vi "template_labview.vi"() -> ()   [LabVIEW 2022 SP3]
uses:
  <vilib>/Utility/file.llb/Write Delimited Spreadsheet (string).vi
  <vilib>/Utility/file.llb/Read Delimited Spreadsheet (string).vi
panel:
  in  "read":bool
  out "all rows":string[][](array[string]) caption="所有行"
  in  "save":bool
  out "数组":string[][](array[string])
  in  "布尔":bool
  in  "数值":i32
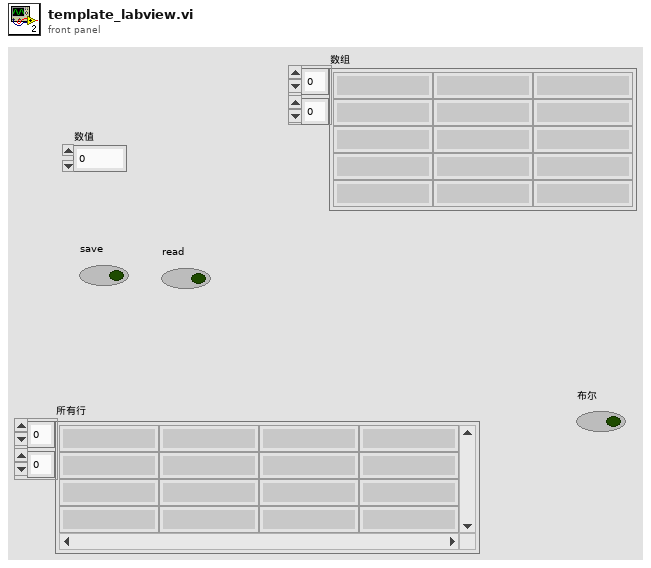
[diagram p1: front panel]
types:
  T1 = cluster{"Number":i32, "Path":path, "Array":string[][]}
  T2 = enum16{"open", "replace", "create", "open or create", "replace or create", "replace or create with confirmation"}
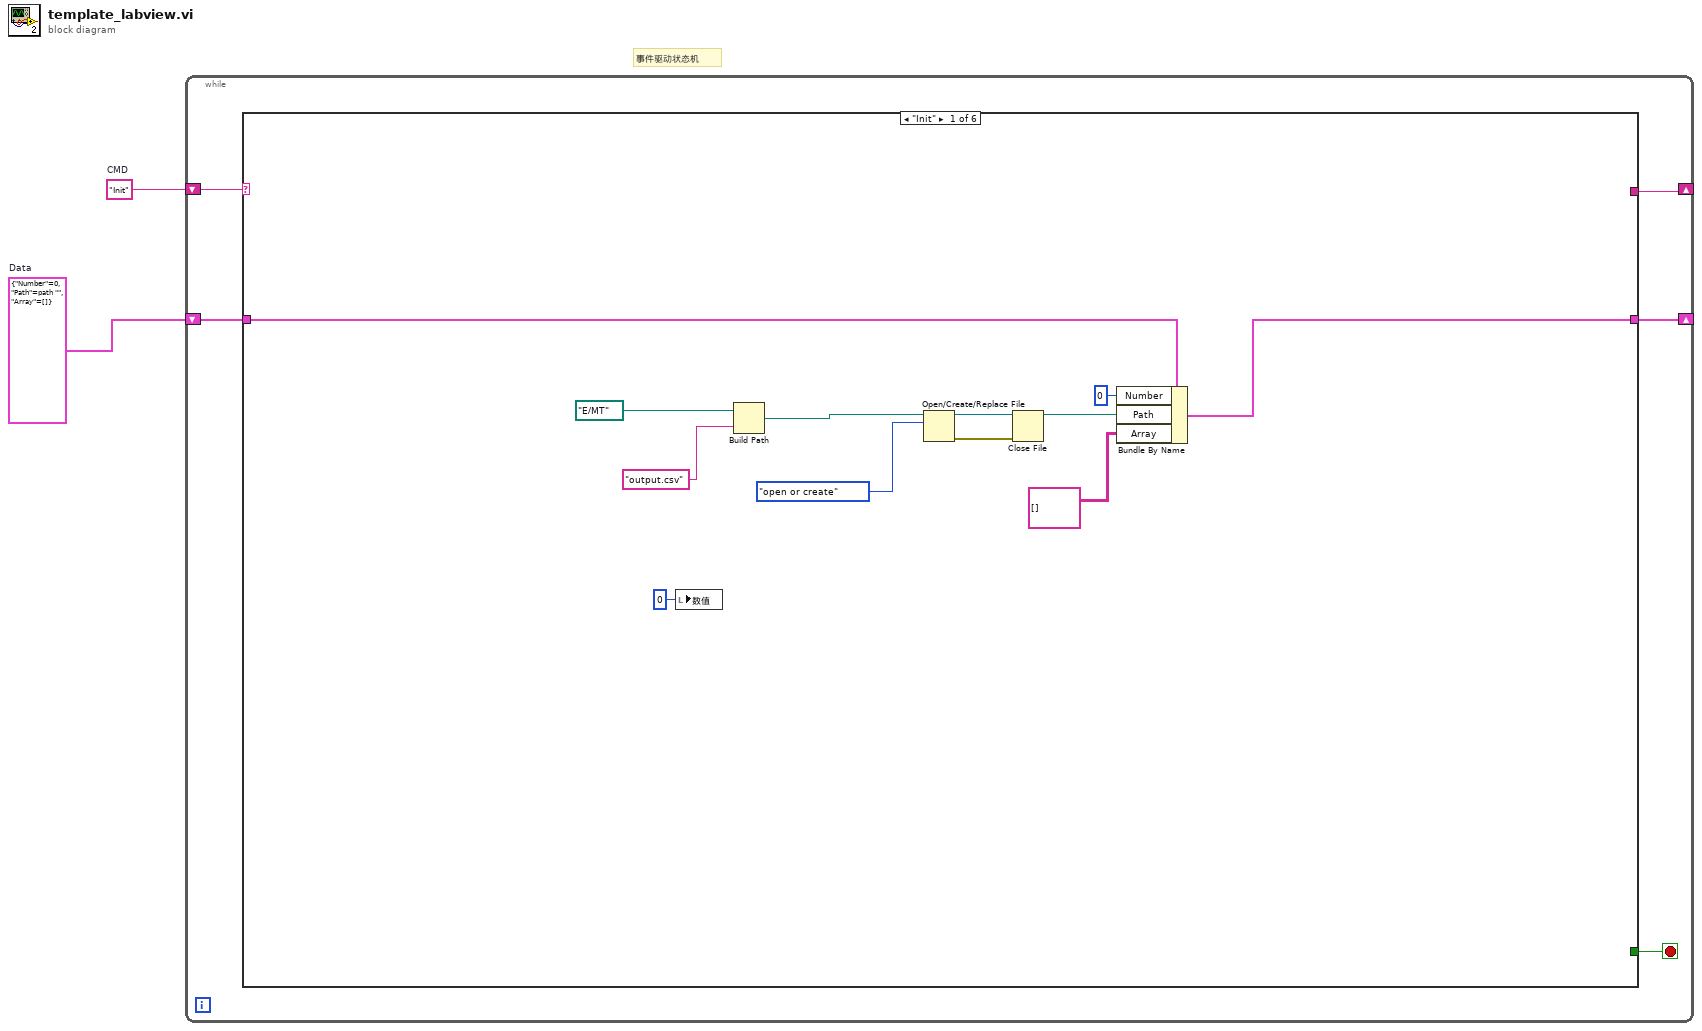
[diagram p0: block diagram]
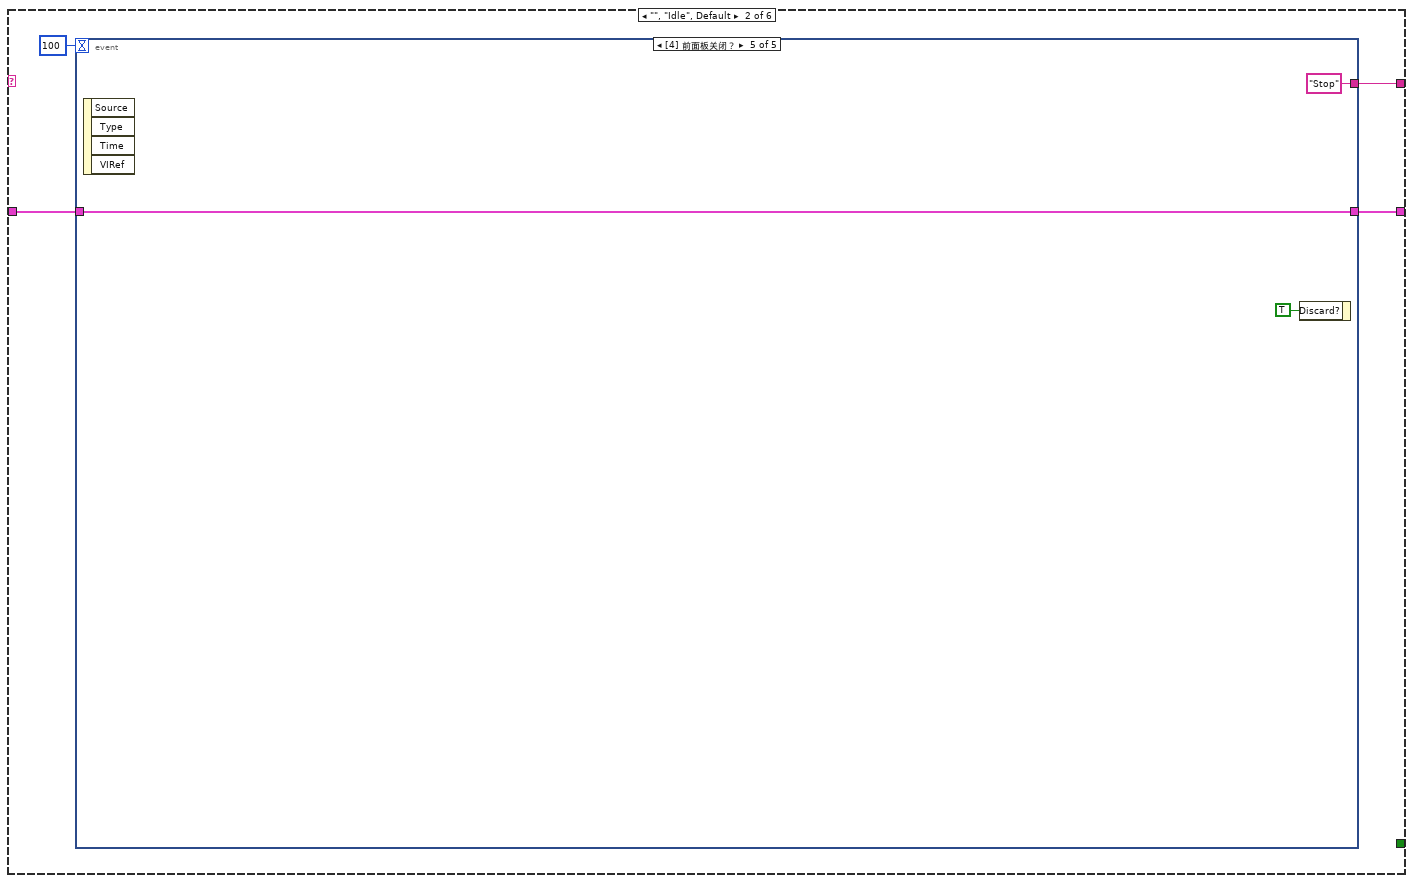
[diagram p2: hidden frame]
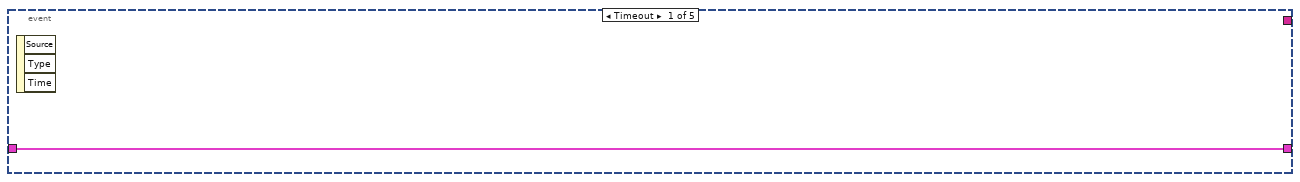
[diagram p3: hidden frame]
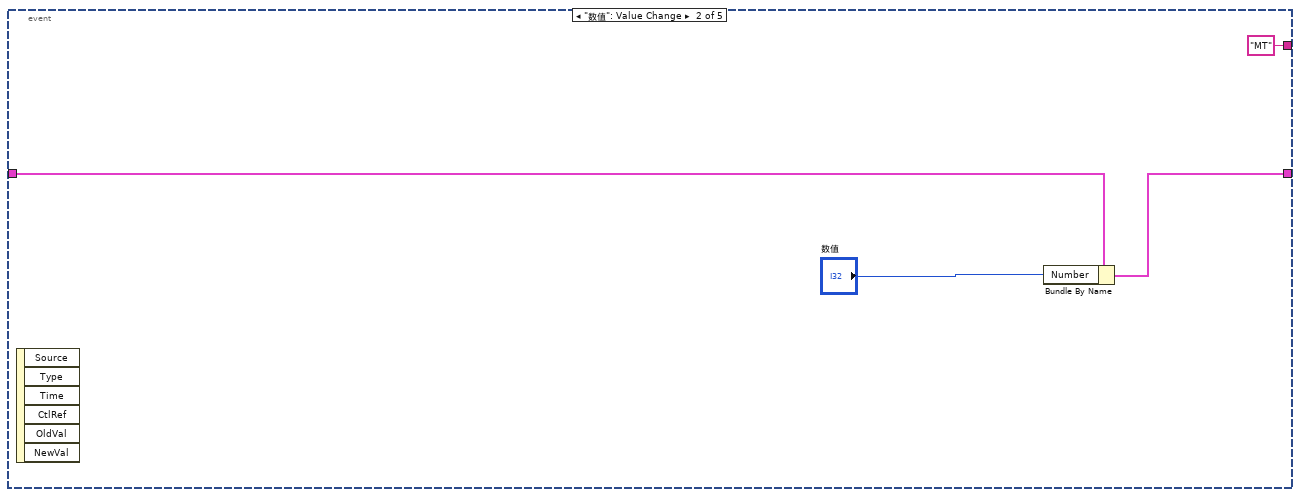
[diagram p4: hidden frame]
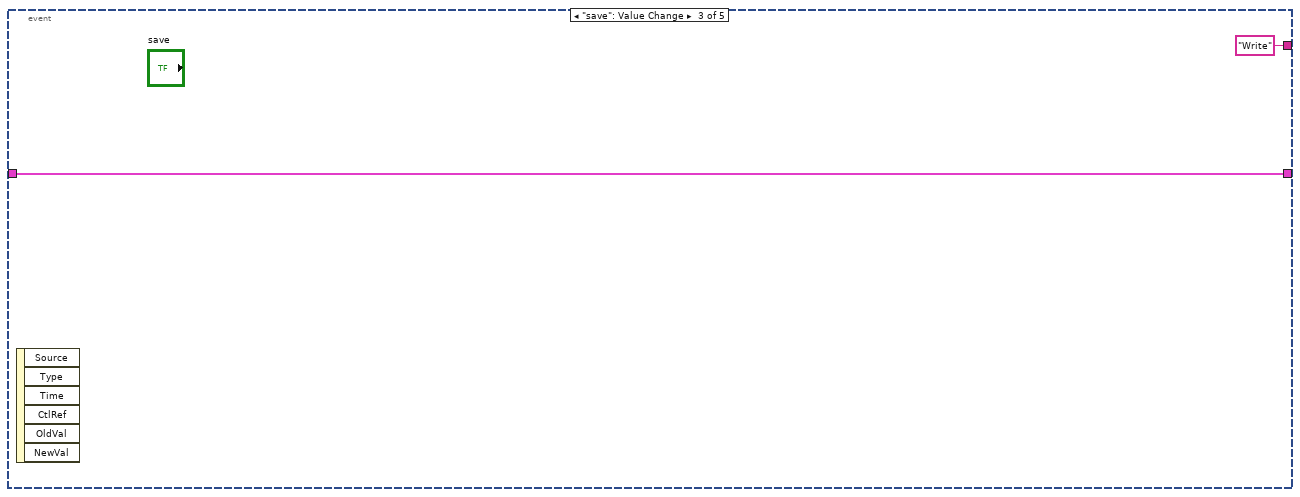
[diagram p5: hidden frame]
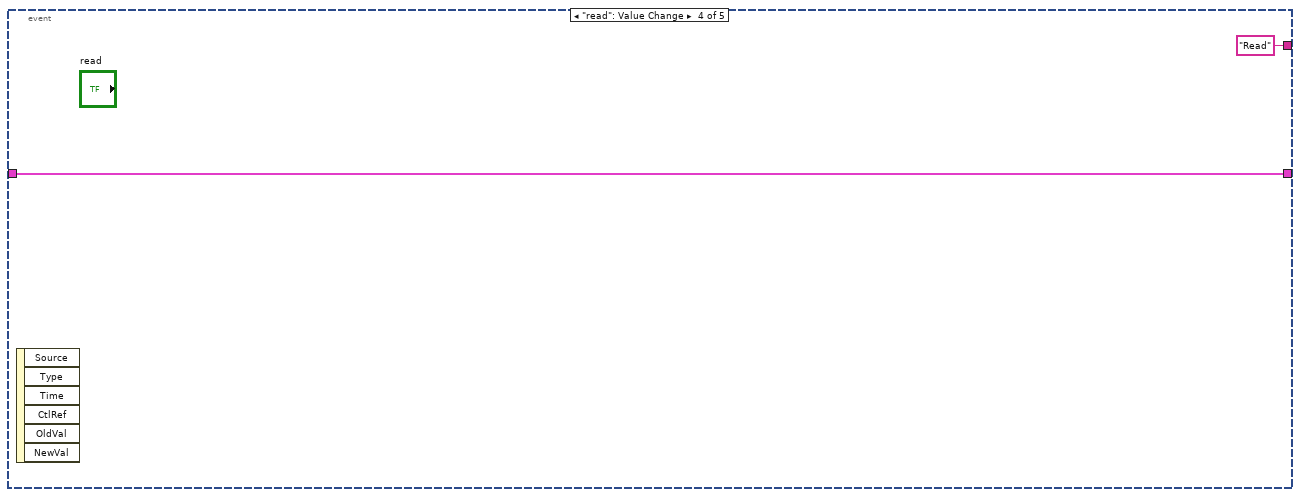
[diagram p6: hidden frame]
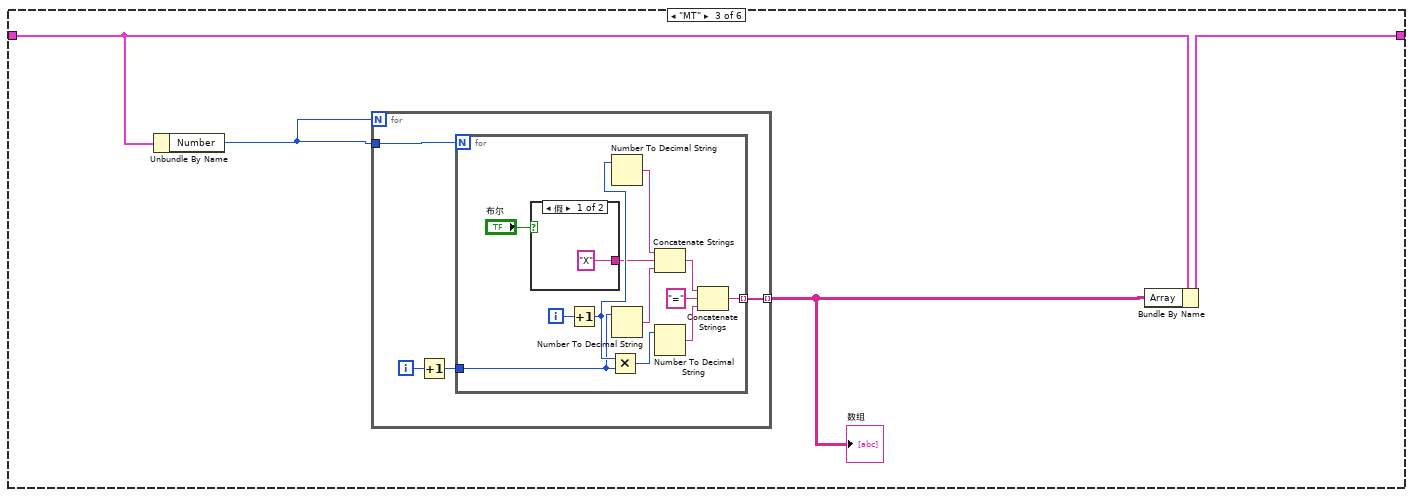
[diagram p7: hidden frame]
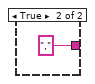
[diagram p8: hidden frame]
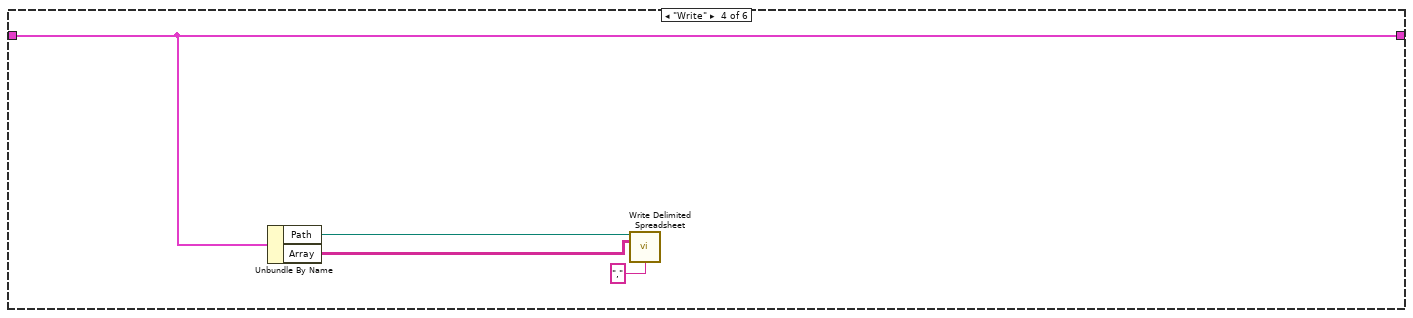
[diagram p9: hidden frame]
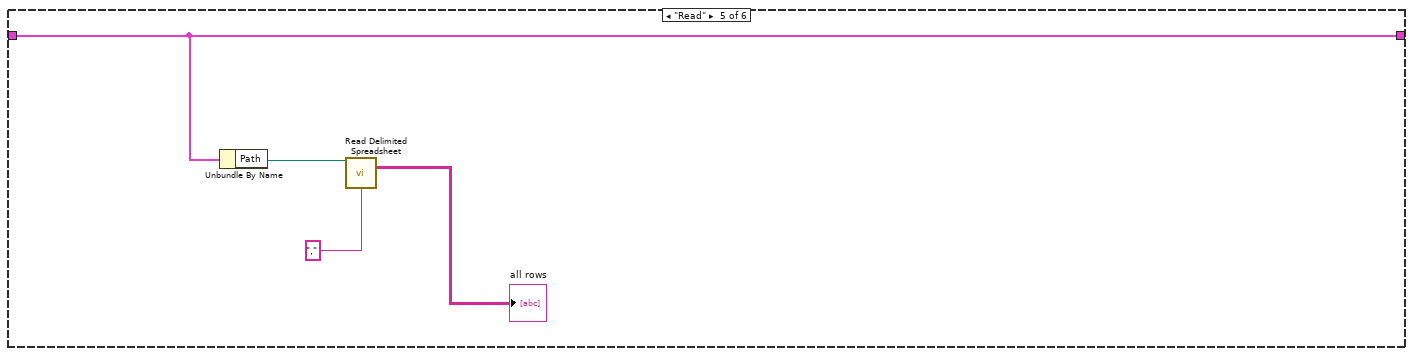
[diagram p10: hidden frame]
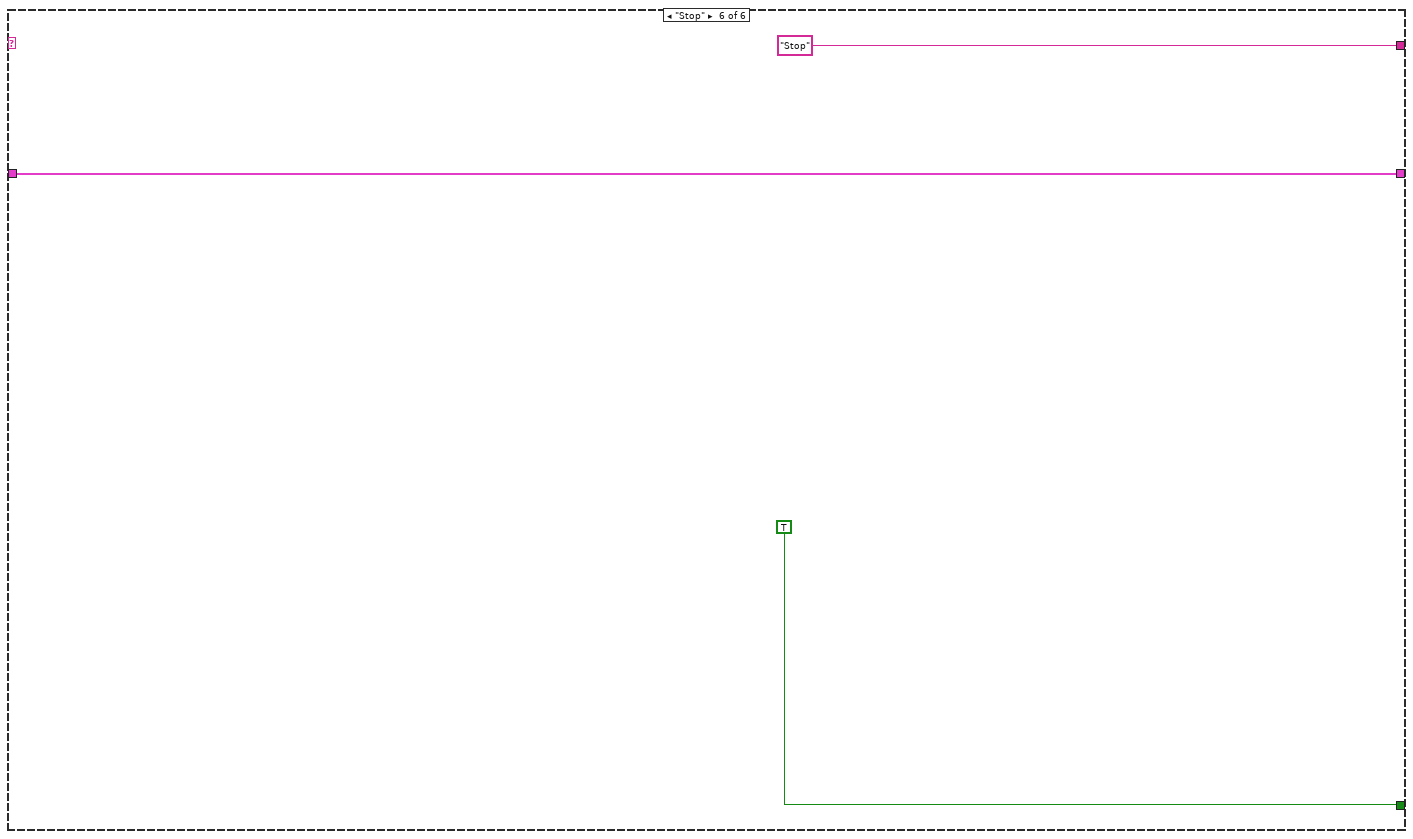
[diagram p11: hidden frame]
diagram:
  w1 = T1 {"Number"=0, "Path"=path "", "Array"=[]}  # Data
  w2 = "Init"  # CMD
  # "事件驱动状态机"
  n1 = while {
    shift-right: [w5] -> _
    shift-left: w2 -> [w7]
    shift-right: [w3] -> _
    shift-left: w1 -> [w4]
    stop <- w6 stop-if-true
    n2 = case shown="\"Init\"" w7 {
      tunnel: [_ _ _ _ _ TRUE] -> w6
      tunnel: [_ w22 _ _ _ "Stop"] -> w5
      tunnel: w4 -> [w19 w21 w39 w60 w65 w66]
      tunnel: [w18 w20 w37 w60 w65 w66] -> w3
      frame "Init" {
        n3 = local write "数值"(0 ("数值")) -> ()
        n4 = Build Path(base path=path "E:/MT" ("Path"), name or relative path="output.csv") -> (appended path=w13:path)
        n5 = Open/Create/Replace File(file path (use dialog)=w13, operation (0:open)=T2."open or create" ("操作(0:open)")) -> (refnum out=w12:refnum<file>, error out=w10:errorcluster)  [unwired: 4 in, 1 out]
        n6 = Close File(refnum=w12, error in=w10) -> (path=w11:path)  [unwired: 1 out]
        n7 = Bundle By Name(cluster=w19, "Number"=0, "Path"=w11, "Array"=string[][] []) -> (w18:T1)
      }
      frame "", "Idle", Default {
        n8 = event shown="[4] 前面板关闭？" {
          selector: _ -> [_ _ _ _ _]
          dyn-events: _ -> [_ _ _ _ _]
          timeout: 100 -> [_ _ _ _ _]
          tunnel: [_ "MT" "Write" "Read" "Stop"] -> w22
          tunnel: w21 -> [w24 w28 w30 w32 w33]
          tunnel: [w24 w27 w30 w32 w33] -> w20
          event Timeout {
            n9 = event-data() -> ()  [unwired: 1 in, 3 out]
          }
          event "数值": Value Change {
            n10 = event-data() -> ()  [unwired: 1 in, 6 out]
            n11 = Bundle By Name(cluster=w28, "Number"="数值") -> (w27:T1)
          }
          event "save": Value Change {
            n12 = event-data() -> ()  [unwired: 1 in, 6 out]
          }
          event "read": Value Change {
            n13 = event-data() -> ()  [unwired: 1 in, 6 out]
          }
          event Panel Close? {
            n14 = event-data() -> ()  [unwired: 1 in, 4 out]
            n15 = event-data("Discard?"=TRUE ("放弃？")) -> ()  [unwired: 1 in, 1 out]
          }
        }
      }
      frame "MT" {
        n16 = Unbundle By Name(w39) -> ("Number"=w38:i32)
        n17 = for {
          N: w38 -> [_]
          tunnel: w38 -> [w43]
          tunnel: [w40] -> w36 mode=indexing
          i -> [w42]
          n18 = Increment(x=w42) -> (x+1=w41:i32)
          n19 = for {
            N: w43 -> [_]
            tunnel: w41 -> [w52]
            tunnel: [w44] -> w40 mode=indexing
            i -> [w54]
            n20 = case shown="假" "布尔" {
              tunnel: ["X" ","] -> w51
              frame False {
              }
              frame True {
              }
            }
            n21 = Increment(x=w54) -> (x+1=w53:i32)
            n22 = Multiply(x=w53, y=w52) -> (x*y=w46:i32)
            n23 = Number To Decimal String(number=w53) -> (decimal integer string=w50:string)  [unwired: 1 in]
            n24 = Number To Decimal String(number=w52) -> (decimal integer string=w49:string)  [unwired: 1 in]
            n25 = Concatenate Strings(w50, w51, w49) -> (w47:string)
            n26 = Number To Decimal String(number=w46) -> (decimal integer string=w45:string)  [unwired: 1 in]
            n27 = Concatenate Strings(w47, "=" ("字符串"), w45) -> (w44:string)
          }
        }
        "数组" <- w36
        n28 = Bundle By Name(cluster=w39, "Array"=w36) -> (w37:T1)
      }
      frame "Write" {
        n29 = Unbundle By Name(w60) -> ("Path"=w59:path, "Array"=w58:string[][])
        n30 = call-poly <vilib>:"Write Delimited Spreadsheet.vi"("file path (dialog if empty)"=w59, "2D data"=w58, "delimiter (\\t)"="," ("delimiter (\\t)")) -> ()  [unwired: 11 in, 2 out]
      }
      frame "Read" {
        n31 = Unbundle By Name(w65) -> ("Path"=w64:path)
        n32 = call-poly <vilib>:"Read Delimited Spreadsheet.vi"("file path (dialog if empty)"=w64, "delimiter (\\t)"="," ("delimiter (\\t)")) -> ("all rows"=→"all rows":string[][])  [unwired: 8 in, 5 out]
      }
      frame "Stop" {
      }
    }
  }
